vi "place sensor on baseplate v2.vi"   [LabVIEW 2020]
uses:
  Classes/Workspace/Pick Up Tool Area/Pick Up Tool Fixture.lvclass
  Classes/Workspace/Component/Component Tray.lvclass
  Classes/Workspace/Carrier Tray/Assembly Tray.lvclass
  Classes/Controller/Controller.lvclass
  Classes/Routine/Pick and Place/Pick and Place.lvclass
  Classes/Routine/Pick and Place/Pick and Place Type.ctl
  Classes/Workspace/Fixture.lvclass
types:
  T1 = typedef "Pick and Place.lvclass/Pick and Place Type.ctl" = enum16{"Primary Pick Up", "Secondary Pick Up", "Put Down All", "Pick Up All", "Put Down Secondary"}
  T2 = typedef "Controller.lvclass/Controllers.ctl" = cluster{"I-O.lvclass":refnum<class "I-O.lvclass">, "Gantry":refnum<k24>, "Dispenser":refnum<visa-resource-name>}
  T3 = typedef "Fixture.lvclass/Workspace.ctl" = cluster{"XYZTheta":dbl[], "Workspace Valve":i32, "Workspace Sensor":i32}
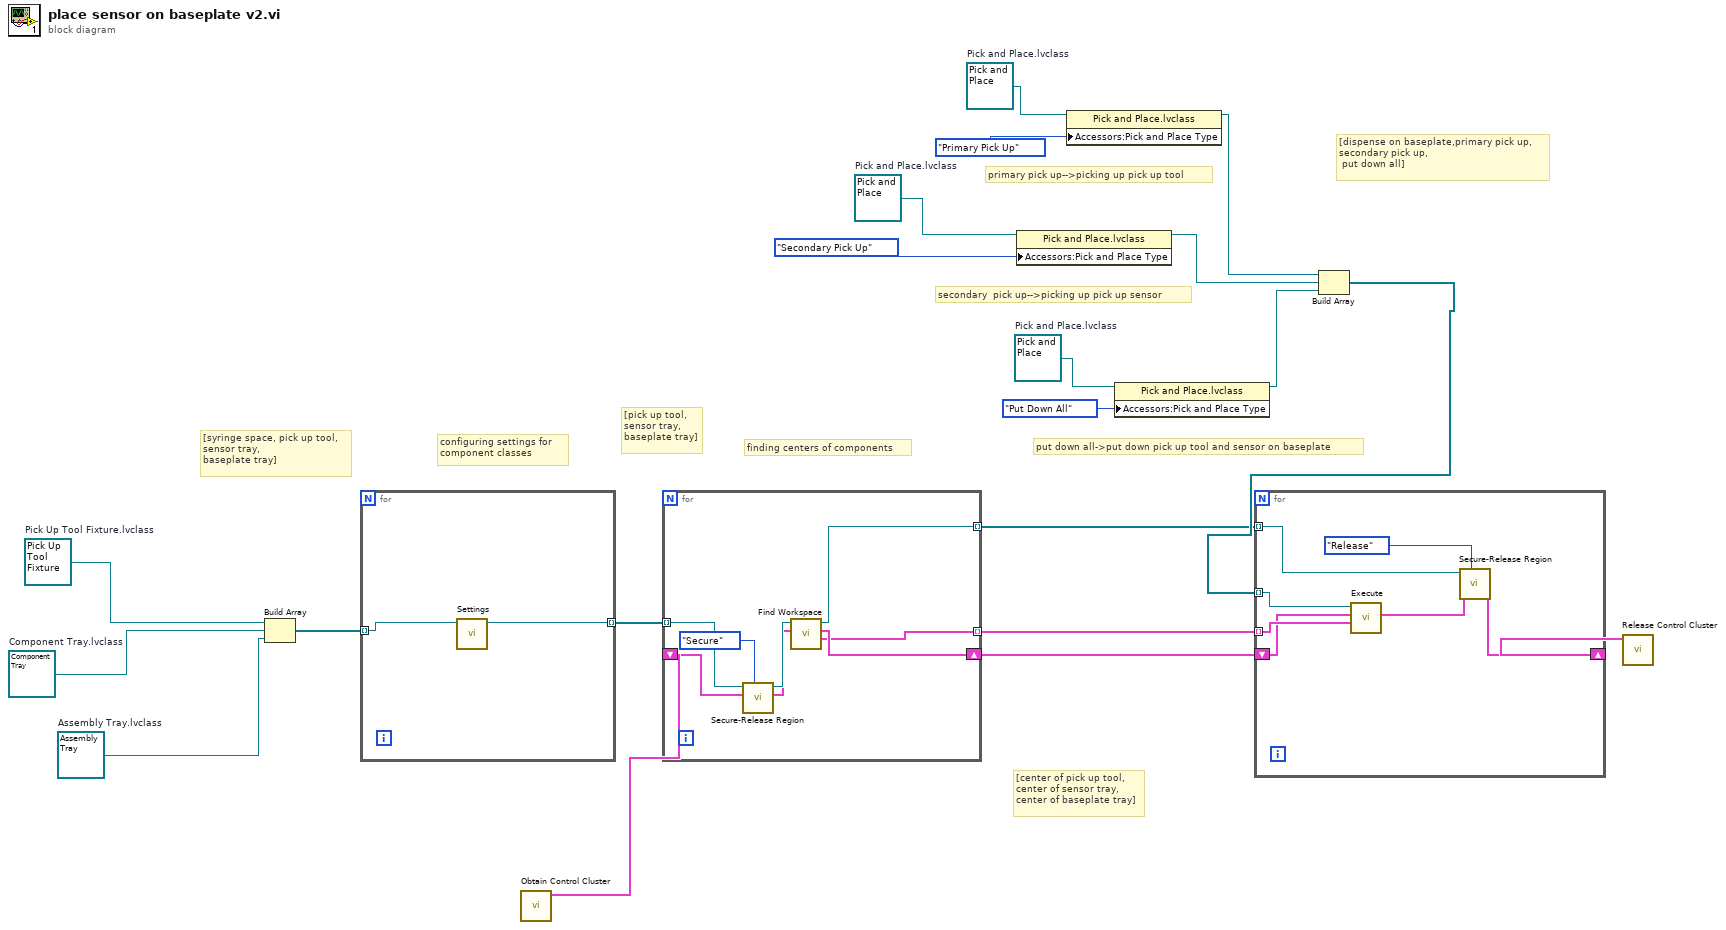
[diagram p0: block diagram]
diagram:
  w10 = refnum<class "Pick and Place.lvclass"> refnum  # Pick and Place.lvclass
  w12 = refnum<class "Pick and Place.lvclass"> refnum  # Pick and Place.lvclass
  w14 = refnum<class "Pick and Place.lvclass"> refnum  # Pick and Place.lvclass
  w18 = refnum<class "Assembly Tray.lvclass"> refnum  # Assembly Tray.lvclass
  w19 = refnum<class "Component Tray.lvclass"> refnum  # Component Tray.lvclass
  w20 = refnum<class "Pick Up Tool Fixture.lvclass"> refnum  # Pick Up Tool Fixture.lvclass
  # "[dispense on baseplate,primary pick up,\nsecondary pick up,\n put down all]"
  # "put down all->put down pick up tool and sensor on baseplate"
  # "secondary  pick up-->picking up pick up sensor"
  # "primary pick up-->picking up pick up tool"
  # "[center of pick up tool,\ncenter of sensor tray,\ncenter of baseplate tray]"
  # "[pick up tool,\nsensor tray,\nbaseplate tray]"
  # "[syringe space, pick up tool,\nsensor tray,\nbaseplate tray]"
  # "finding centers of components"
  # "configuring settings for \ncomponent classes"
  n1 = Build Array(w20, w19, w18) -> (w17:refnum<class "Fixture.lvclass">[])
  n2 = for {
    tunnel: w17 -> [w22] mode=indexing
    tunnel: [w21] -> w16 mode=indexing
    n3 = call-dynamic "Settings.vi"("Workspace in"=w22) -> ("Workspace out"=w21:refnum<class "Fixture.lvclass">)  [unwired: 9 in, 1 out]
  }
  n4 = call "Obtain Control Cluster.vi"() -> ("Control Out"=w15:T2)  [unwired: 11 in]
  n5 = for {
    tunnel: w16 -> [w28] mode=indexing
    shift-right: [w30] -> w3
    shift-left: w15 -> [w26]
    tunnel: [w29] -> w4 mode=indexing
    tunnel: [w23] -> w1 mode=indexing
    n6 = call-dynamic "Secure-Release Region.vi"("Action"=enum16{"Secure", "Release"}."Secure", "Control In"=w26, "Fixture in"=w28) -> ("Control Out"=w25:T2, "Fixture out"=w27:refnum<class "Fixture.lvclass">)  [unwired: 6 in, 1 out]
    n7 = call-dynamic "Find Workspace.vi"("Control In"=w25, "Workspace In"=w27) -> (1:"Workspace Out"=w29:T3, "Control Out"=w30:T2, 3:"Workspace Out"=w23:refnum<class "Fixture.lvclass">)  [unwired: 6 in, 1 out]
  }
  n8 = property class="Pick and Place.lvclass"(reference=w12, "Accessors:Pick and Place Type"=Pick_and_Place_Type."Secondary Pick Up" ("Pick and Place Type")) -> (reference out=w7:refnum<class "Pick and Place.lvclass">)  [unwired: 1 in, 1 out]
  n9 = property class="Pick and Place.lvclass"(reference=w14, "Accessors:Pick and Place Type"=Pick_and_Place_Type."Primary Pick Up" ("Pick and Place Type")) -> (reference out=w8:refnum<class "Pick and Place.lvclass">)  [unwired: 1 in, 1 out]
  n10 = property class="Pick and Place.lvclass"(reference=w10, "Accessors:Pick and Place Type"=Pick_and_Place_Type."Put Down All" ("Pick and Place Type")) -> (reference out=w6:refnum<class "Pick and Place.lvclass">)  [unwired: 1 in, 1 out]
  n11 = Build Array(w8, w7, w6) -> (w5:refnum<class "Pick and Place.lvclass">[])
  n12 = for {
    tunnel: w5 -> [w37] mode=indexing
    tunnel: w4 -> [w36] mode=indexing
    shift-right: [w33] -> w2
    shift-left: w3 -> [w35]
    tunnel: w1 -> [w32] mode=indexing
    n13 = call-dynamic "Execute.vi"("Workspace"=w36, "Cluster"=w35, "Pick and Place in"=w37) -> ("Control Out"=w34:T2)  [unwired: 6 in, 2 out]
    n14 = call-dynamic "Secure-Release Region.vi"("Action"=enum16{"Secure", "Release"}."Release", "Control In"=w34, "Fixture in"=w32) -> ("Control Out"=w33:T2)  [unwired: 6 in, 2 out]
  }
  n15 = call "Release Control Cluster.vi"("output cluster"=w2) -> ()  [unwired: 11 in]
